vi "ErrorDetector.vi"(10 "Data":T3, 11 "User Input":T2) -> (3 "Cluster":T1)   [LabVIEW 2017]
uses:
  Ctrl/Data.ctl
  Ctrl/Caps.ctl
  Ctrl/Property.ctl
  Ctrl/PhysicalChannel.ctl
  Ctrl/Register.ctl
  Ctrl/Bitfield.ctl
  Ctrl/Scale.ctl
  Ctrl/ScaleType.ctl
  Ctrl/Enum.ctl
  Ctrl/EnumValue.ctl
  Ctrl/UserInput.ctl
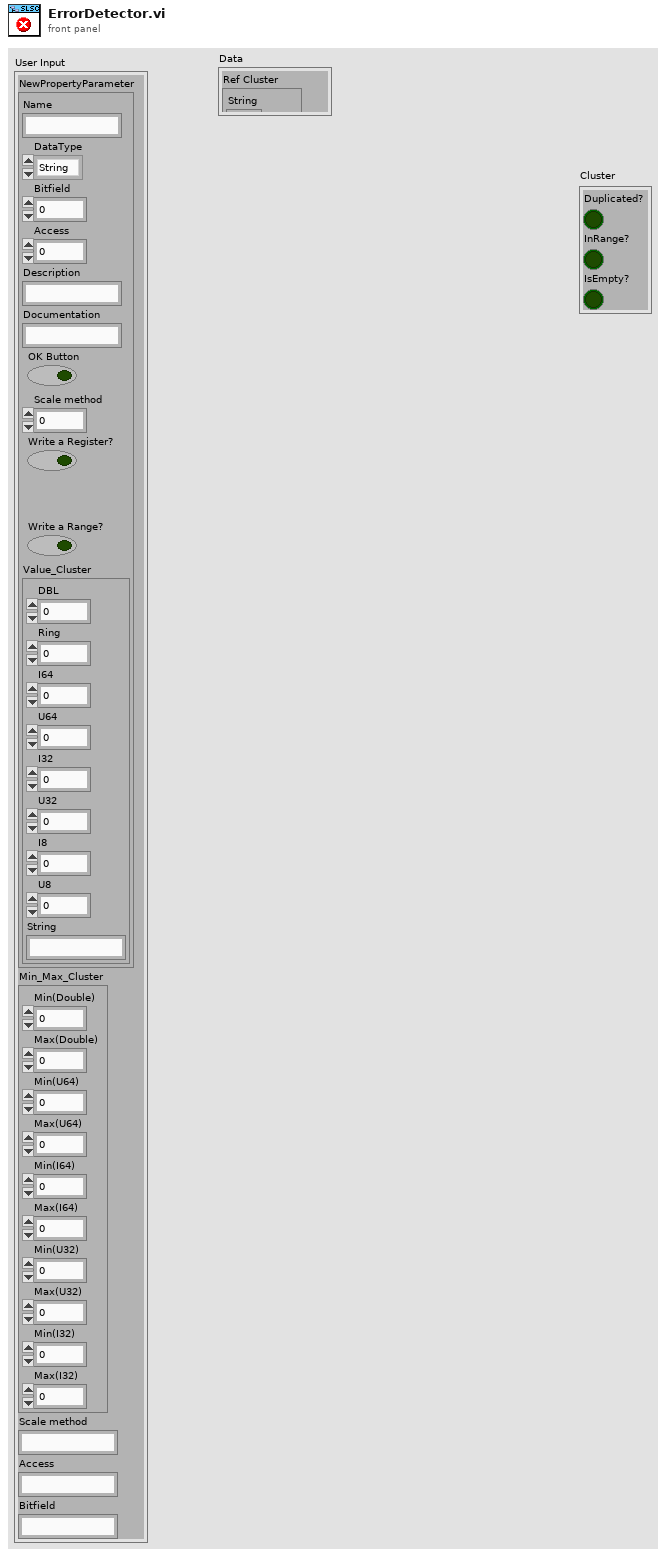
[diagram p1: front panel]
types:
  T1 = cluster{"Duplicated?":bool, "InRange?":bool, "IsEmpty?":bool}
  T2 = typedef "UserInput.ctl" = cluster{"NewPropertyParameter":cluster{"Name":string, "DataType":enum16{"String", "Double", "U64", "I64", "U32", "I32", "Bool"}, "Bitfield":u16, "Access":u16, "Description":string, "Documentation":string, "OK Button":bool, "Scale method":u16, "Write a Register?":bool, "Write a Range?":bool, "Value_Cluster":cluster{"DBL":dbl, "Ring":u16, "I64":i64, "U64":u64, "I32":i32, "U32":u32, "I8":i8, "U8":u8, "String":string}}, "Min_Max_Cluster":cluster{"Min(Double)":dbl, "Max(Double)":dbl, "Min(U64)":u64, "Max(U64)":u64, "Min(I64)":i64, "Max(I64)":i64, "Min(U32)":u32, "Max(U32)":u32, "Min(I32)":i32, "Max(I32)":i32}, "Scale method":string, "Access":string, "Bitfield":string}
  T3 = typedef "Data.ctl" = cluster{"Ref Cluster":cluster{"String":refnum<vi>, "U8":refnum<vi>, "I8":refnum<vi>, "U32":refnum<vi>, "I32":refnum<vi>, "U64":refnum<vi>, "I64":refnum<vi>, "Ring":refnum<vi>, "DBL":refnum<vi>, "Add":refnum<vi>, "Remove":refnum<vi>, "Property tree":refnum<vi>, "confirm":refnum<vi>}, "JSON Text":string, "Original JSON Text":string, "Caps":T4, "SLSC Output Tree":cluster{"Left Cell String":string, "Child Text":string[], "Child Tag":string, "Item Indent":i32, "Child Only?":bool, "Glyph Index":i32, "offline value":variant}[], "Ref Index and Control Type":cluster{"index":i32, "Datatype":string}, "Selected Type and name":cluster{"Selected Type":enum16{"Property", "Physical Channel", "Other"}, "Selected Property Name":string}, "Update whole Tree?":bool}
  T4 = typedef "Caps.ctl" = cluster{"properties":T5[], "physical channels":T6[], "registers":T7[], "scales":T9[], "enums":T11[], "productName":string}
  T5 = typedef "Property.ctl" = cluster{"name":string, "bitfield":string, "value":variant, "dataType":string, "min":variant, "max":variant, "scale":string, "access":string}
  T6 = typedef "PhysicalChannel.ctl" = cluster{"name":string, "properties":T5[]}
  T7 = typedef "Register.ctl" = cluster{"name":string, "address":i32, "size":i32, "bitfields":T8[], "initialValue":variant, "connectedProperties":string[]}
  T8 = typedef "Bitfield.ctl" = cluster{"name":string, "offset":i32, "size":i32, "signed":bool}
  T9 = typedef "Scale.ctl" = cluster{"name":string, "type":T10, "params":variant}
  T10 = typedef "ScaleType.ctl" = enum16{"NoScale", "Table", "Polynomial", "Linear"}
  T11 = typedef "Enum.ctl" = cluster{"name":string, "values":T12[]}
  T12 = typedef "EnumValue.ctl" = cluster{"name":string, "value":i32}
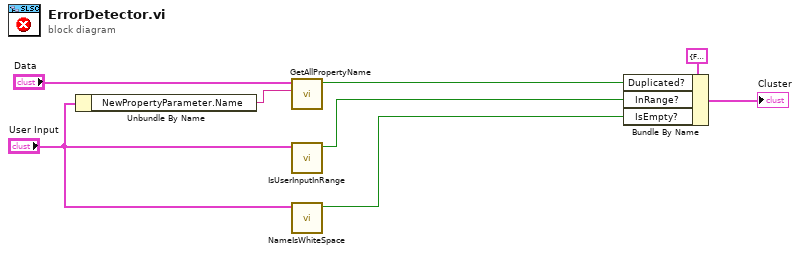
[diagram p0: block diagram]
diagram:
  n1 = Unbundle By Name("User Input") -> ("NewPropertyParameter.Name"=w7:string)
  n2 = call "GetAllPropertyName.vi"("NewPropertyName"=w7, "Data"="Data") -> ("Duplicated Name?"=w6:bool)  [unwired: 9 in]
  n3 = call "IsUserInputInRange.vi"("User Input in"="User Input") -> ("InRange?"=w5:bool)  [unwired: 10 in]
  n4 = call "NameIsWhiteSpace.vi"("User Input"="User Input") -> ("IsWhiteSpaceOrEmpty?"=w4:bool)  [unwired: 10 in]
  n5 = Bundle By Name(cluster=T1 {"Duplicated?"=FALSE, "InRange?"=TRUE, "IsEmpty?"=FALSE} ("Cluster"), "Duplicated?"=w6, "InRange?"=w5, "IsEmpty?"=w4) -> (→"Cluster":T1)
